vi "Grouped_Proj _newa_steploop_FINAL.vi"() -> ()   [LabVIEW 2017]
uses:
  <instrlib>/Lake Shore 336/Public/Data/Sensor Data (Single Reading).vi
  <vilib>/Utility/file.llb/Write Delimited Spreadsheet (DBL).vi
  <instrlib>/Lake Shore 336/Lake Shore 336.lvlib
panel:
  in  "Temp tolerance":dbl
  in  "Temp end":dbl
  in  "step":dbl
  in  "Temp start":dbl
  in  "stop":bool
  in  "Heater Range":u16(ring) items=["Off", "Low (On)", "Medium", "High"]
  in  "Rate (D) (0.0 %)":dbl format="%.1f"
  in  "Reset (I) (20.0)":dbl=20.0 format="%.1f"
  in  "Gain (P) (50.0)":dbl=50.0 format="%.1f"
  in  "Input (0:None)":u16(ring) items=["None", "A", "B", "C", "D"]
  in  "Output's Control Loop (1:1)":u16(ring)=1 items=["1"=1, "2"=2]
  out "Measured Temperature":dbl format="%.4g"
  in  "Temperature controller address":refnum<visa-resource-name>
  in  "file to save data (dialog if empty)":path
  in  "Resistance Range Lower Limit (2 Ohm)":dbl=2.0 format="%#_6p"
  in  "Resistance Range Upper Limit (2E+8 Ohm)":dbl=200000000.0 format="%#_6p"
  in  "Resistance NPLC (0.1)":dbl=0.1
  in  "Resistance Range (2 Ohm)":dbl=2.0
  in  "Resistance Auto Range (T: Enable)":bool=TRUE
  out "Measured Resistance (Ohms)":dbl format="%#_6p"
  in  "Source Meter address":refnum<visa-resource-name>="GPIB1::29::INSTR"
  in  "Error In":errorcluster
  # "Resistance vs Temperature Measurement"
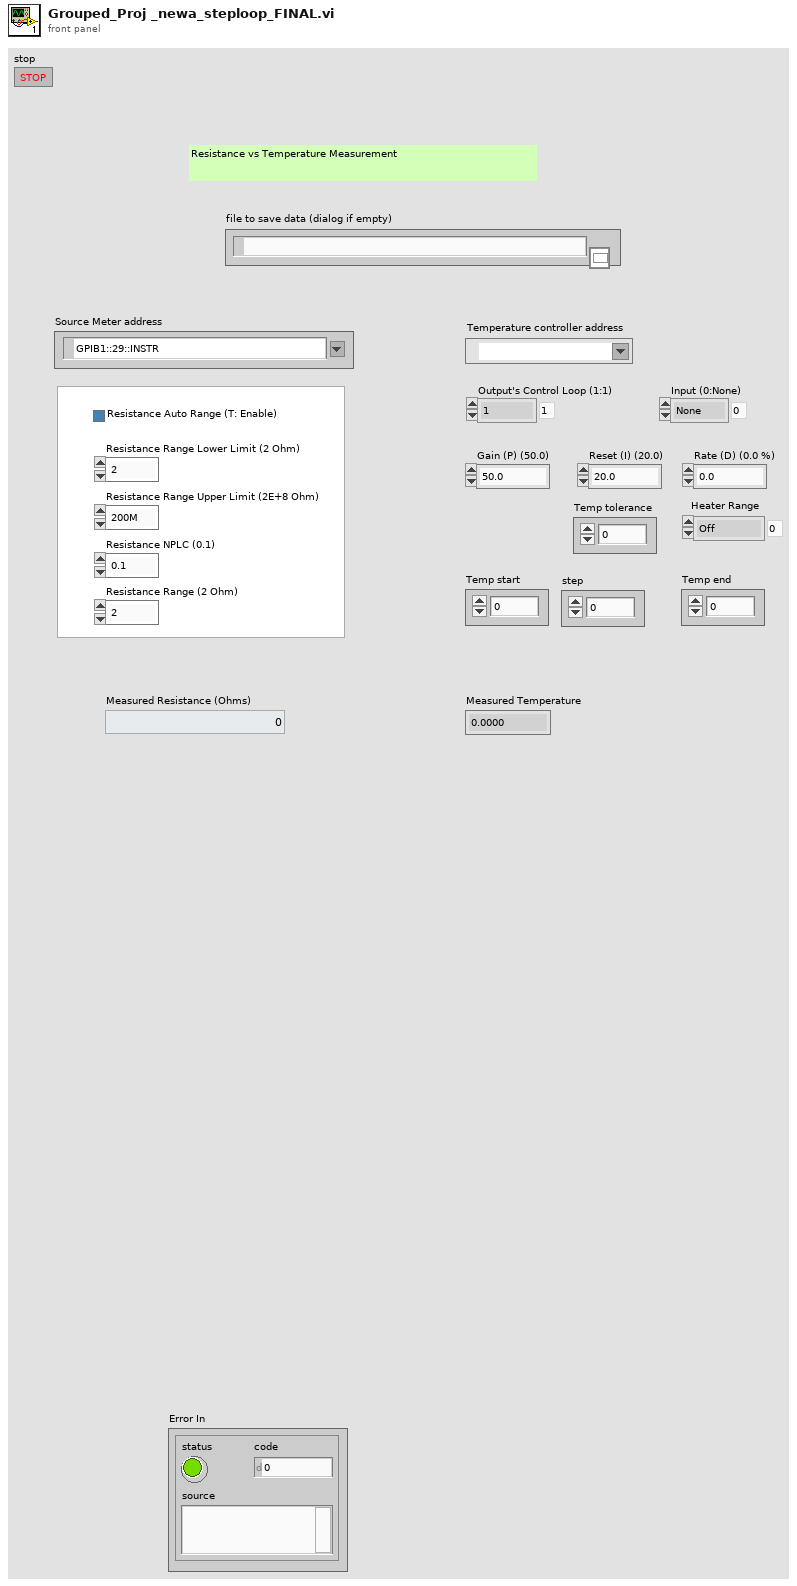
[diagram p1: front panel]
types:
  T1 = cluster{"Baud Rate":u32, "Parity":u16, "Data Bits":u16, "Stop Bits":u16, "Flow Control":u16}
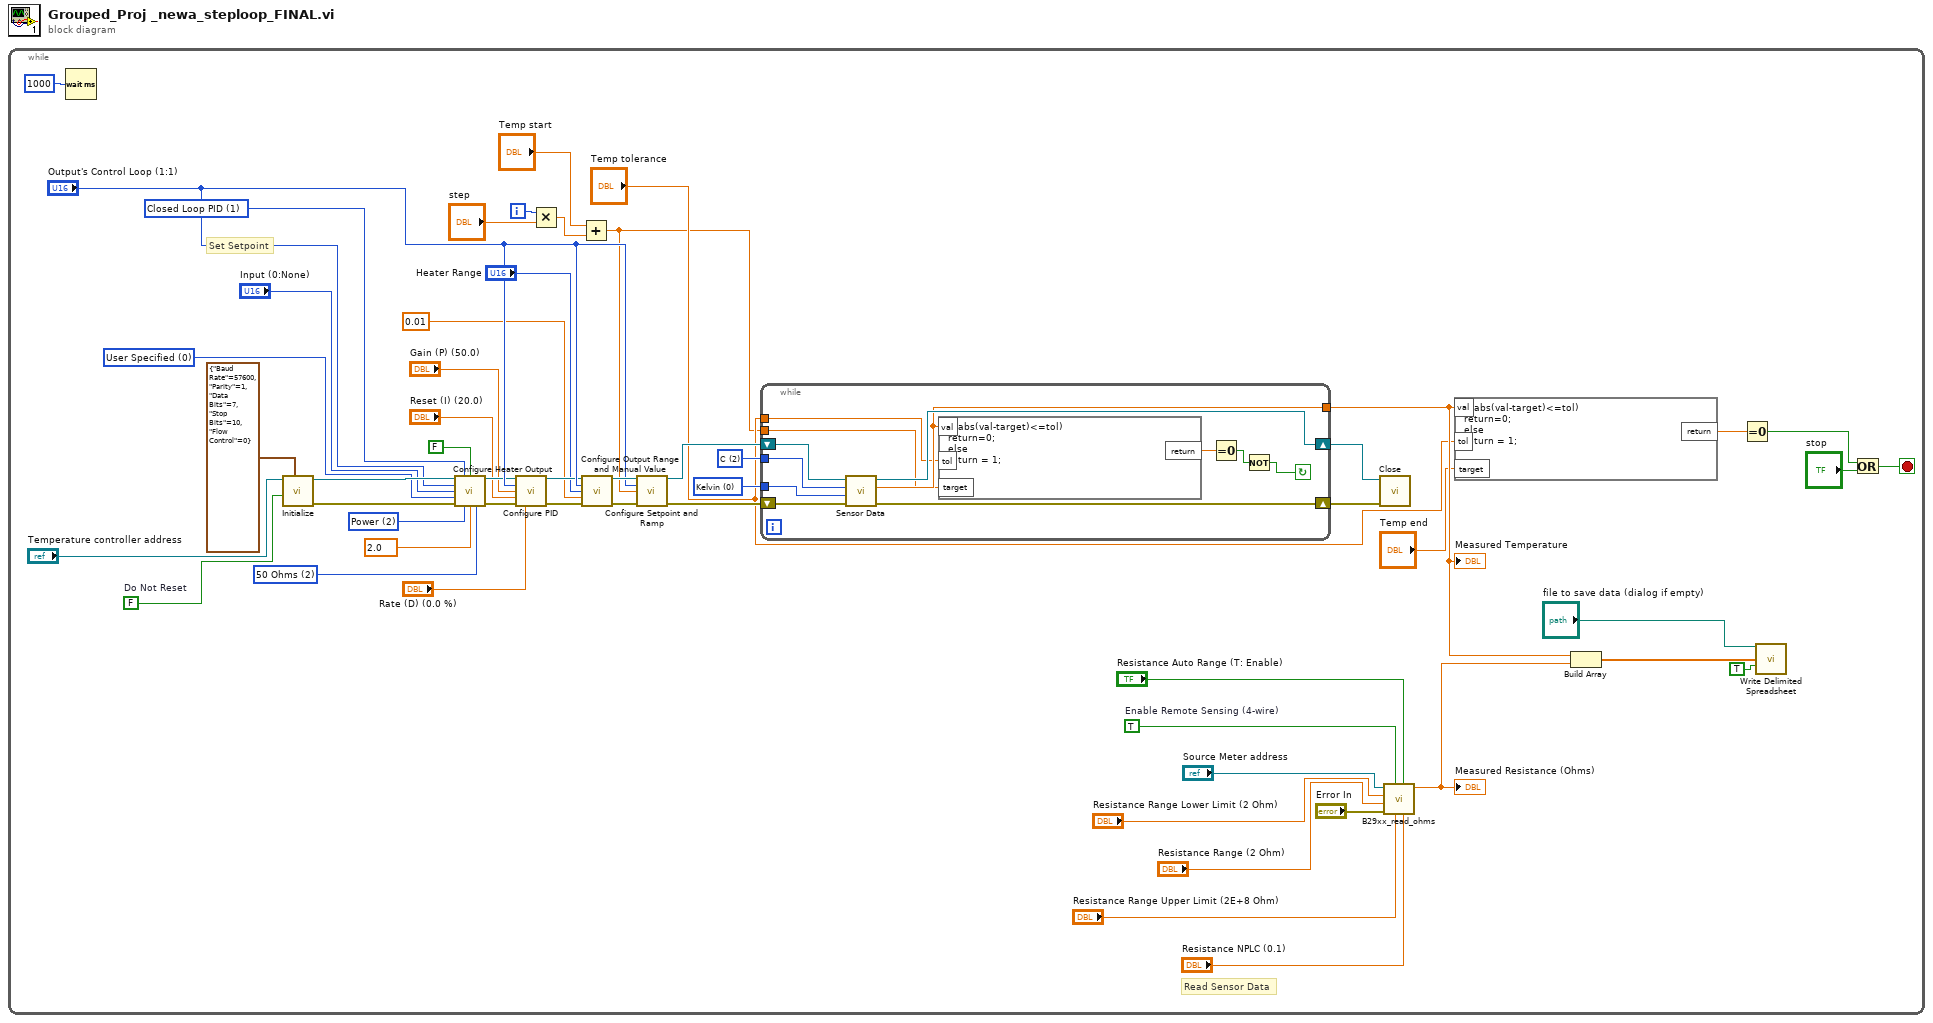
[diagram p0: block diagram]
diagram:
  n1 = while {
    i -> [w5]
    stop <- w11 stop-if-true
    w24 = u16 0 items=["User Specified", "0.707 A", "1.0 A", "1.141 A", "2.0 A"] ("Max Current (0:User Specified)")
    w25 = u16 1 items=["Off", "Closed Loop PID", "Zone", "Open Loop"] ("Mode (0:Off)")
    w14 = u16 2 items=["A", "B", "C", "D"] ("Input (0:A)")
    w21 = u16 2 items=["50 Ohms"=2, "25 Ohms"=1] ("Heater Resistance (default to 50Ohms)")
    w34 = u16 0 items=["Kelvin", "Celsius", "Sensor Units"] ("Data Source (0:Kelvin)")
    w23 = u16 2 items=["Current"=1, "Power"=2] ("Heater Out Display (1:Current)")
    w38 = FALSE  # Do Not Reset
    w53 = TRUE  # Enable Remote Sensing (4-wire)
    # "Set Setpoint"
    # "Read Sensor Data"
    n2 = Wait (ms)(milliseconds to wait=u32 1000) -> ()  [unwired: 1 out]
    n3 = call <instrlib>:"Initialize.vi"("Serial Configuration"=T1 {"Baud Rate"=57600, "Parity"=1, "Data Bits"=7, "Stop Bits"=10, "Flow Control"=0}, "Reset (True)"=w38, "VISA resource name"="Temperature controller address") -> ("error out"=w42:errorcluster, "VISA resource name out"=w43:refnum<visa-resource-name>)  [unwired: 7 in]
    n4 = call <instrlib>:"Configure Heater Output.vi"("VISA resource name"=w43, "Mode (0:Off)"=w25, "Power Up Enable (F: Off)"=FALSE, "Heater Output (1:1)"="Output's Control Loop (1:1)", "Input (0:None)"="Input (0:None)", "Max Current (0:User Specified)"=w24, "error in (no error)"=w42, "Heater Out Display (1:Current)"=w23, "Max User Current (2.000)"=2.0, "Heater Resistance (1:25 Ohms)"=w21) -> ("VISA resource name out"=w29:refnum<visa-resource-name>, "error out"=w30:errorcluster)  [unwired: 4 in]
    n5 = call <instrlib>:"Configure PID.vi"("VISA resource name"=w29, "Output's Control Loop (1:1)"="Output's Control Loop (1:1)", "Gain (P) (50.0)"="Gain (P) (50.0)", "Reset (I) (20.0)"="Reset (I) (20.0)", "error in (no error)"=w30, "Rate (D) (0.0 %)"="Rate (D) (0.0 %)") -> ("VISA resource name out"=w28:refnum<visa-resource-name>, "error out"=w27:errorcluster)  [unwired: 8 in]
    n6 = Multiply(x=w5, y="step") -> (x*y=w3:dbl)
    n7 = Add(x="Temp start", y=w3) -> (x+y=w1:dbl)
    n8 = call <instrlib>:"Configure Output Range and Manual Value.vi"("VISA resource name"=w28, "Output (1:1)"="Output's Control Loop (1:1)", "Range (0:Off)"="Heater Range", "Manual Output (0.00 %)"=0.01, "error in (no error)"=w27) -> ("VISA resource name out"=w40:refnum<visa-resource-name>, "error out"=w39:errorcluster)  [unwired: 9 in]
    n9 = call <instrlib>:"Configure Setpoint and Ramp.vi"("VISA resource name"=w40, "Output's Control Loop (1:1)"="Output's Control Loop (1:1)", "Setpoint (0.00000)"=w1, "error in (no error)"=w39) -> ("VISA resource name out"=w36:refnum<visa-resource-name>, "error out"=w35:errorcluster)  [unwired: 10 in]
    n10 = while {
      tunnel: w34 -> [w65]
      tunnel: w14 -> [w62]
      tunnel: [w60] -> w8
      shift-right: [w64] -> w33
      shift-left: w36 -> [w67]
      shift-right: [w63] -> w32
      shift-left: w35 -> [w66]
      tunnel: "Temp tolerance" -> [w59]
      tunnel: w1 -> [w58]
      stop <- w56 continue-if-true
      n11 = call-poly <instrlib>:"Sensor Data.vi"("error in (no error)"=w66, "Data Source (0:Kelvin)"=w65, "Input (0:A)"=w62, "VISA resource name"=w67) -> ("error out"=w63:errorcluster, "Sensor Data"=w60:dbl, "VISA resource name out"=w64:refnum<visa-resource-name>)  [unwired: 5 in]
      n12 = formula code="if(abs(val-target)<=tol)\nreturn=0;\nelse \nreturn = 1;"("val"=w60, "tol"=w59, "target"=w58) -> ("return"=w61:dbl)
      n13 = Equal To 0?(x=w61) -> (x = 0?=w57:bool)
      n14 = Not(x=w57) -> (.not. x?=w56:bool)
    }
    "Measured Temperature" <- w8
    n15 = call <instrlib>:"Close.vi"("error in (no error)"=w32, "VISA resource name"=w33) -> ()  [unwired: 9 in, 1 out]
    n16 = call "B29xx_read_ohms.vi"("Resistance NPLC (0.1)"="Resistance NPLC (0.1)", "Resistance Auto Range (T: Enable)"="Resistance Auto Range (T: Enable)", "Resistance Range Upper Limit (2E+8 Ohm)"="Resistance Range Upper Limit (2E+8 Ohm)", "Enable Remote Sensing (4-wire)"=w53, "error in (no error)"="Error In", "Resistance Range (2 Ohm)"="Resistance Range (2 Ohm)", "Resistance Range Lower Limit (2 Ohm)"="Resistance Range Lower Limit (2 Ohm)", "VISA Refnum in"="Source Meter address") -> ("Measurement Result"=w44:dbl)  [unwired: 2 in, 1 out]
    "Measured Resistance (Ohms)" <- w44
    n17 = formula code="if(abs(val-target)<=tol)\nreturn=0;\nelse \nreturn = 1;"("val"=w8, "tol"="Temp tolerance", "target"="Temp end") -> ("return"=w9:dbl)
    n18 = Build Array(w8, w44) -> (w46:dbl[])
    n19 = Equal To 0?(x=w9) -> (x = 0?=w10:bool)
    n20 = call-poly <vilib>:"Write Delimited Spreadsheet.vi"("file path (dialog if empty)"="file to save data (dialog if empty)", "1D data"=w46, "append to file? (new file:F)"=TRUE) -> ()  [unwired: 11 in, 2 out]
    n21 = Or(x=w10, y="stop") -> (x .or. y?=w11:bool)
  }
